vi "Periodic Tasks.vi"(8 "error in":errorcluster) -> ()   [LabVIEW 2015]
doc: "This VI runs in parallel to other tasks. It can contain as many user-defined periodic loops as you need. These can carry out PID or other sorts of timed response."
uses:
  <vilib>/Rock Robotics/Network Tables/NT Write Boolean.vi
  Robot Global Data.vi
  <vilib>/Rock Robotics/Network Tables/NT Write Numeric Array.vi
  <vilib>/Rock Robotics/Network Tables/NT Read Boolean.vi
  <vilib>/Rock Robotics/Network Tables/NT Write Number.vi
  <vilib>/Rock Robotics/SystemInterfaces/AI/FPGA_AIChannel.ctl
  Team900-VIs/navX Library v2/navX Library v2.lvlib
panel:
  out "Distance":bool
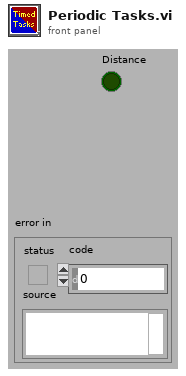
[diagram p1: front panel]
types:
  T1 = typedef "FPGA_AIChannel.ctl" = enum8{"AI 0", "AI 1", "AI 2", "AI 3", "AI MXP 0", "AI MXP 1", "AI MXP 2", "AI MXP 3", "Invalid"}
  T2 = typedef "WPI_AnalogChannelDevRef.ctl" = cluster{"DevStatus":errorcluster, "Analog Channel":T1}
  T3 = typedef "navX Library v2.lvlib/Z900_navX_DeviceTypeDef.ctl" = cluster{"Interface":cluster{"Protocol":T4, "Update Rate (4Hz-60Hz)":u8, "navX Open TypeDef":variant}, "Notify Packet":refnum<notifier>, "Loop VI Refnum":refnum<vi>, "Ready to Close Occurrence Refnum":refnum<k4>}
  T4 = typedef "navX Library v2.lvlib/Z900_navX_ProtocolTypeDef.ctl" = enum16{"SERIAL", "I2C", "SPI"}
  T5 = cluster{"Yaw":dbl, "Roll":dbl, "Pitch":dbl, "Heading":dbl, "Fused Heading":dbl}
  T6 = typedef "WPI_MotorControlDeviceRef.ctl" = cluster{"DeviceStatus":errorcluster, "Type":T7, "PWM":cluster{"PWM Channel":T8, "DeadBand":T9}, "CAN":cluster{"Device Number":u8, "Control Mode":T10, "Semaphore":T11, "Max Vout":dbl, "TalonSRX Control Mode":T12}, "Invert":bool}
  T7 = typedef "WPI_MotorControlType.ctl" = enum16{"PWM", "CAN", "CANTalonSRX"}
  T8 = typedef "FPGA_DIOPWMChannel.ctl" = enum8{"PWM 0", "PWM 1", "PWM 2", "PWM 3", "PWM 4", "PWM 5", "PWM 6", "PWM 7", "PWM 8", "PWM 9", "PWM MXP 0", "PWM MXP 1", "PWM MXP 2", "PWM MXP 3", "PWM MXP 4", "PWM MXP 5", "PWM MXP 6", "PWM MXP 7", "PWM MXP 8", "PWM MXP 9", "Invalid"}
  T9 = typedef "WPI_PWMDeadband.ctl" = cluster{"Name":string, "maxPositivePwm":i32, "minPositivePwm":i32, "centerPwm":i32, "maxNegativePwm":i32, "minNegativePwm":i32, "angularRange":u16}
  T10 = typedef "WPI_CANJaguar_ControlMode.ctl" = enum8{"Percent VBus", "Current", "Speed", "Position", "Voltage"}
  T11 = typedef "Semaphore RefNum" = refnum<k1>
  T12 = typedef "WPI_CANTalonSRX_APIControlMode.ctl" = enum8{"Percent VBus", "Speed", "Position", "Slave", "Unchanged / Invalid", "Voltage Compensation", "Current", "Motion Profile"}
  T13 = typedef "WPI_CANTalonSRX_GlobalStatus.ctl" = cluster{"Applied Throttle":dbl, "Module Enabled":bool, "CAN Error":errorcluster, "Closed Loop Error":dbl, "Forward Limit Switch Closed":bool, "Reverse Limit Switch Closed":bool, "Sensor Position":dbl, "Sensor Velocity":dbl, "Current":dbl, "Sticky Fault - Over Temp":bool, "Sticky Fault - Under Voltage":bool, "Sticky Fault - Forward Limit":bool, "Sticky Fault - Reverse Limit":bool, "Sticky Fault - Forward Soft Limit":bool, "Sticky Fault - Reverse Soft Limit":bool, "Brake is Enabled":bool, "Encoder Position":dbl, "Encoder Velocity":dbl, "Encoder Index Count":dbl, "Encoder A Pin State":bool, "Encoder B Pin State":bool, "Encoder Index Pin State":bool, "Analog In":dbl, "Analog In Velocity":dbl, "Temperature (C)":dbl, "Battery Voltage":dbl, "Control 5 Is Supported":bool, "Current Profile Slot Select":dbl, "Pos Div 8":bool, "Vel Div 4":bool, "Pulse Width Position":i32, "Pulse Width Velocity":i32, "Pulse Width Rise To Rise (us)":i32, "Pulse Width Rise To Fall (us)":i32, "Mot Prof Active Is Under Run":bool, "Mot Prof Active Has Under Run":bool, "Mot Prof Active Is Last":bool, "Mot Prof Active Velocity Only":bool, "Mot Prof Active Is Valid":bool, "Mot Prof Buffer Is Full":bool, "Mot Prof Active Profile Slot Select":i32, "Mot Prof NextID":i32, "Mot Prof Count":i32, "Mot Prof Active Velocity":dbl, "Mot Prof Active Position":dbl, "Mot Prof Output Enable":i32}
  T14 = typedef "WPI_DigitalInputDevRef.ctl" = cluster{"DevStatus":errorcluster, "DIO Channel":T15}
  T15 = typedef "FPGA_DIOChannel.ctl" = enum8{"DIO 0", "DIO 1", "DIO 2", "DIO 3", "DIO 4", "DIO 5", "DIO 6", "DIO 7", "DIO 8", "DIO 9", "DIO MXP 0", "DIO MXP 1", "DIO MXP 2", "DIO MXP 3", "DIO MXP 4", "DIO MXP 5", "DIO MXP 6", "DIO MXP 7", "DIO MXP 8", "DIO MXP 9", "DIO MXP 10", "DIO MXP 11", "DIO MXP 12", "DIO MXP 13", "DIO MXP 14", "DIO MXP 15", "Invalid"}
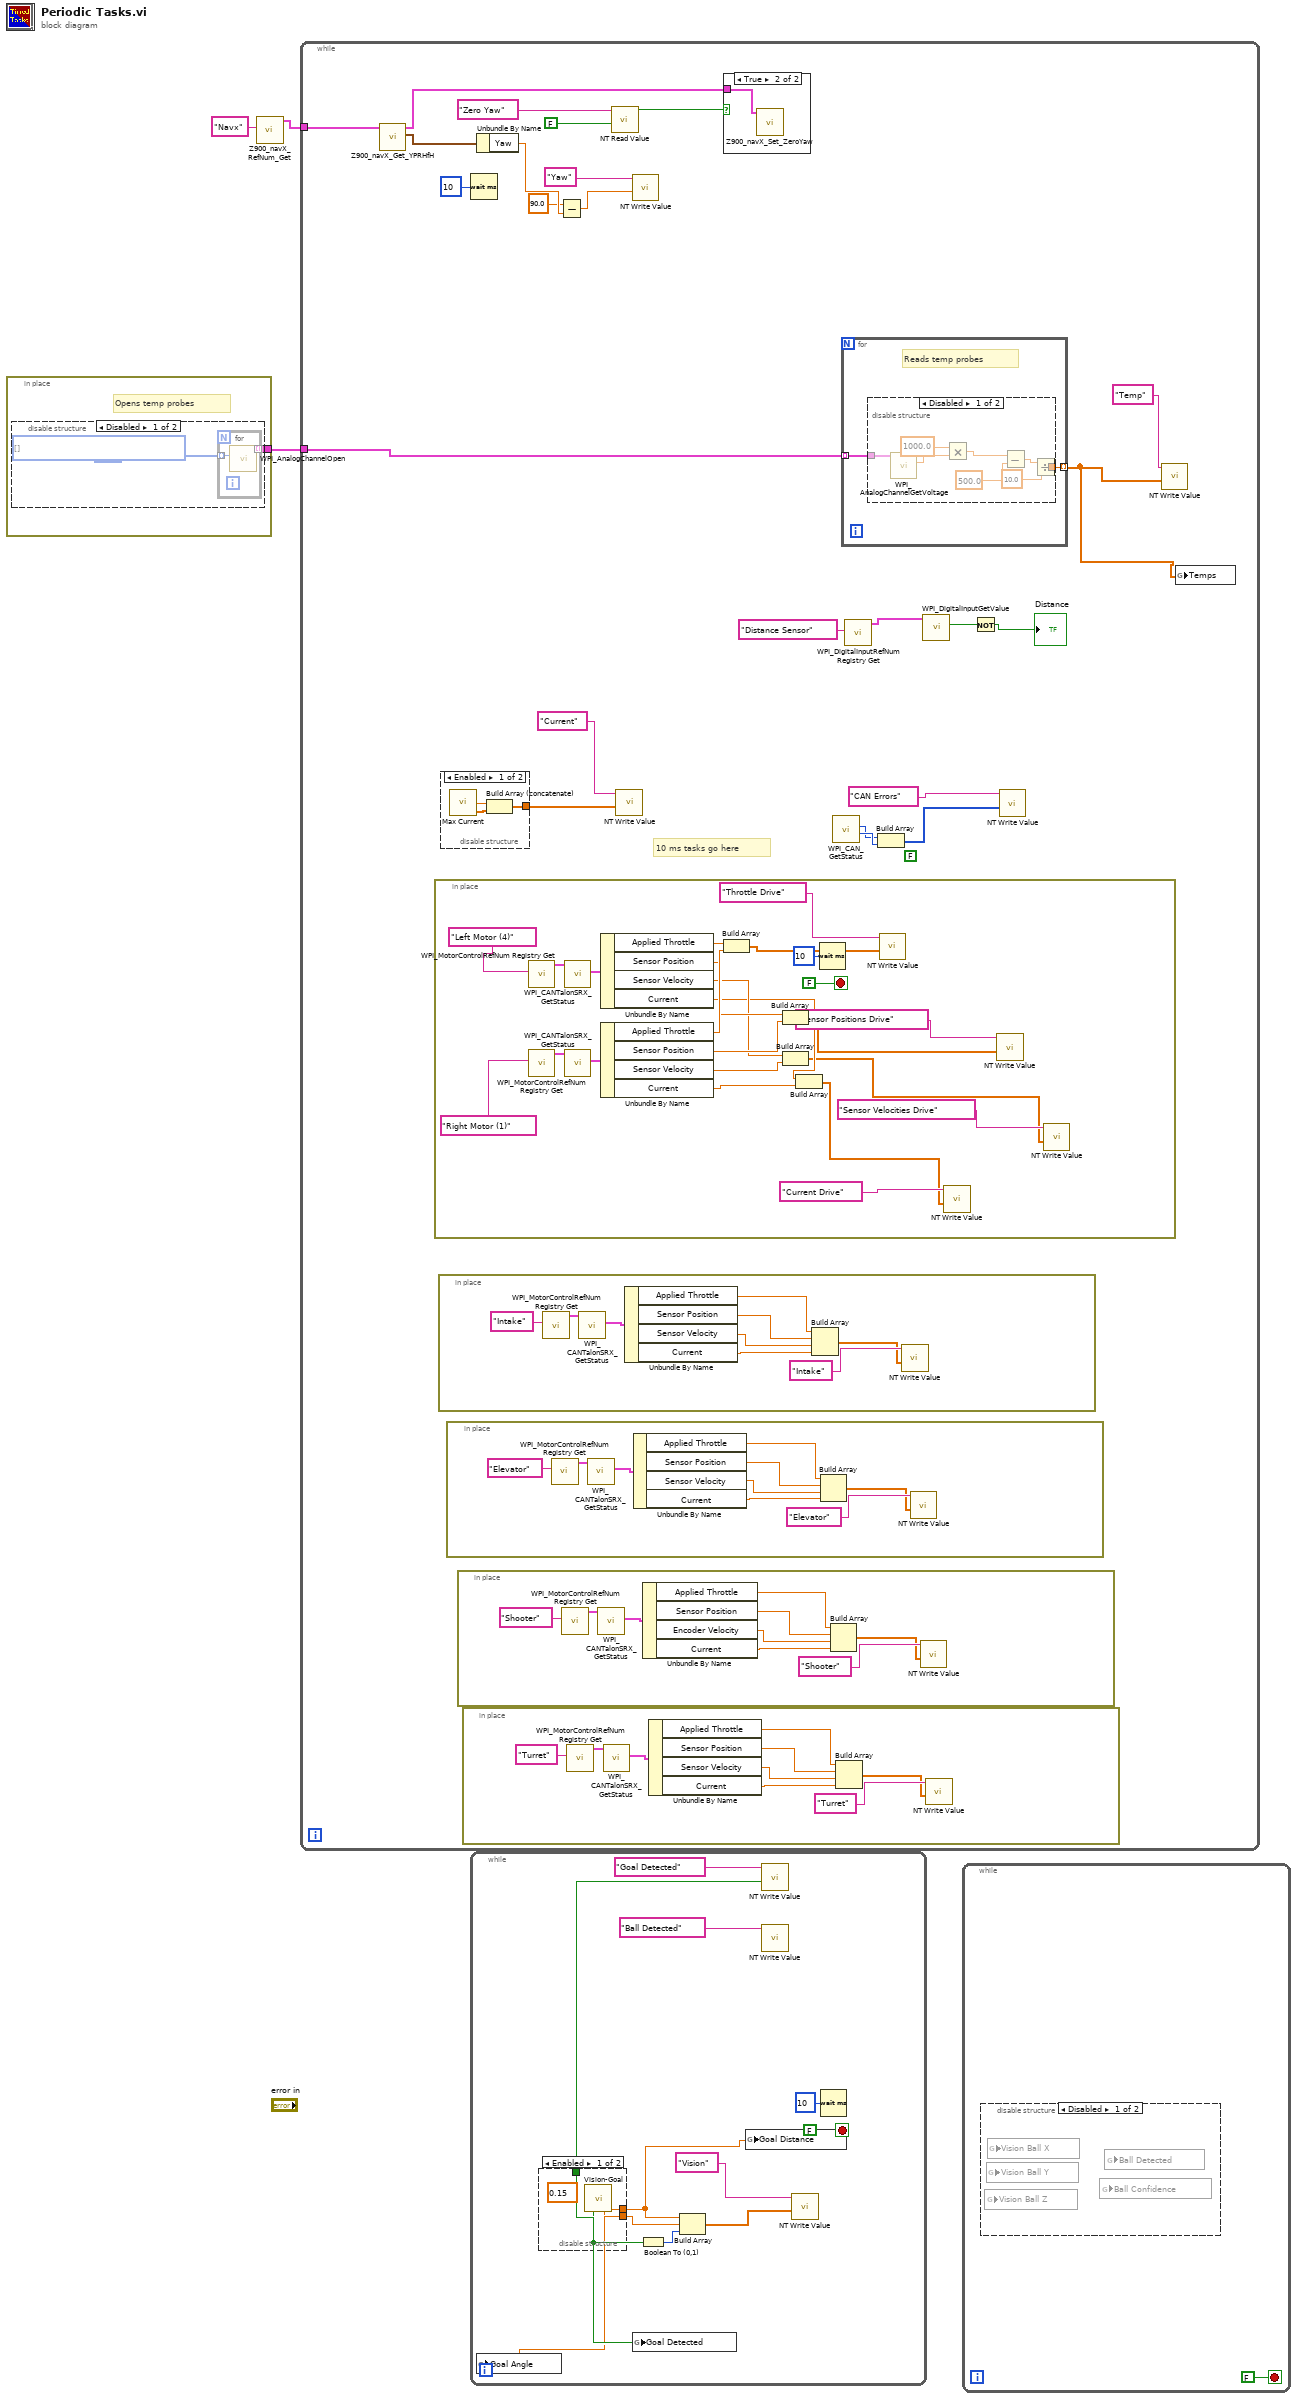
[diagram p0: block diagram]
diagram:
  n1 = in-place {
    in-place-border: [w4] -> w3
    # "Opens temp probes"
    n2 = disable-structure shown="Disabled" {
      disable-tunnel: [w5 _] -> w4
      frame Disabled {
        w6 = T1[] [] items=["AI 0", "AI 1", "AI 2", "AI 3", "AI MXP 0", "AI MXP 1", "AI MXP 2", "AI MXP 3", "Invalid"] ("Analog Channel")
        n3 = for {
          tunnel: w6 -> [w8] mode=indexing
          tunnel: [w7] -> w5 mode=indexing
          n4 = call <vilib>:"WPI_AnalogChannelOpen.vi"("Analog Channel"=w8) -> ("AIDeviceRef"=w7:T2)  [unwired: 9 in, 1 out]
        }
      }
      frame Enabled {
      }
    }
  }
  n5 = call "Z900_navX_RefNum_Get.vi"("refnum name"="Navx") -> ("navX Device"=w1:T3)  [unwired: 9 in, 1 out]
  n6 = while {
    tunnel: w3 -> [w14]
    tunnel: w1 -> [w20]
    stop <- FALSE stop-if-true
    (unwired) FALSE
    # "10 ms tasks go here"
    n7 = call "Z900_navX_Get_YPRHfH.vi"("navX Device"=w20) -> ("YRPHfH"=w19:T5, "navX Device"=w18:T3)  [unwired: 7 in, 2 out]
    n8 = in-place {
      n9 = call <vilib>:"WPI_MotorControlRefNum Registry Get.vi"("refnum name"="Left Motor (4)") -> ("MotorControlDevRef"=w101:T6)  [unwired: 9 in, 1 out]
      n10 = call <vilib>:"WPI_MotorControlRefNum Registry Get.vi"("refnum name"="Right Motor (1)") -> ("MotorControlDevRef"=w102:T6)  [unwired: 9 in, 1 out]
      n11 = call <vilib>:"WPI_CANTalonSRX_GetStatus.vi"("CAN Talon SRX Ref"=w101) -> ("Talon SRX Status"=w99:T13)  [unwired: 8 in, 2 out]
      n12 = call <vilib>:"WPI_CANTalonSRX_GetStatus.vi"("CAN Talon SRX Ref"=w102) -> ("Talon SRX Status"=w100:T13)  [unwired: 8 in, 2 out]
      n13 = Unbundle By Name(w99) -> ("Applied Throttle"=w98:dbl, "Sensor Position"=w96:dbl, "Sensor Velocity"=w94:dbl, "Current"=w91:dbl)
      n14 = Unbundle By Name(w100) -> ("Applied Throttle"=w97:dbl, "Sensor Position"=w95:dbl, "Sensor Velocity"=w93:dbl, "Current"=w92:dbl)
      n15 = Build Array(w98, w97) -> (w89:dbl[])
      n16 = Build Array(w96, w95) -> (w87:dbl[])
      n17 = Build Array(w94, w93) -> (w85:dbl[])
      n18 = Build Array(w91, w92) -> (w83:dbl[])
      n19 = call-poly <vilib>:"NT Write Value.vi"("Numeric Array"=w89, "Name"="Throttle Drive") -> ()  [unwired: 9 in, 1 out]
      n20 = call-poly <vilib>:"NT Write Value.vi"("Numeric Array"=w83, "Name"="Current Drive") -> ()  [unwired: 9 in, 1 out]
      n21 = call-poly <vilib>:"NT Write Value.vi"("Numeric Array"=w87, "Name"="Sensor Positions Drive") -> ()  [unwired: 9 in, 1 out]
      n22 = call-poly <vilib>:"NT Write Value.vi"("Numeric Array"=w85, "Name"="Sensor Velocities Drive") -> ()  [unwired: 9 in, 1 out]
    }
    n23 = in-place {
      n24 = call <vilib>:"WPI_MotorControlRefNum Registry Get.vi"("refnum name"="Intake") -> ("MotorControlDevRef"=w79:T6)  [unwired: 9 in, 1 out]
      n25 = call <vilib>:"WPI_CANTalonSRX_GetStatus.vi"("CAN Talon SRX Ref"=w79) -> ("Talon SRX Status"=w78:T13)  [unwired: 8 in, 2 out]
      n26 = Unbundle By Name(w78) -> ("Applied Throttle"=w77:dbl, "Sensor Position"=w76:dbl, "Sensor Velocity"=w75:dbl, "Current"=w74:dbl)
      n27 = Build Array(w77, w76, w75, w74) -> (w72:dbl[])
      n28 = call-poly <vilib>:"NT Write Value.vi"("Numeric Array"=w72, "Name"="Intake") -> ()  [unwired: 9 in, 1 out]
    }
    n29 = disable-structure shown="Enabled" {
      disable-tunnel: [w103 _] -> w27
      frame Enabled {
        n30 = call "Max Current.vi"() -> ("Currents By Channel"=w104:dbl[], "Current"=w105:dbl)  [unwired: 1 out]
        n31 = Build Array (concatenate)(w105, w104) -> (w103:dbl[])
      }
      frame Disabled {
      }
    }
    n32 = in-place {
      n33 = call <vilib>:"WPI_MotorControlRefNum Registry Get.vi"("refnum name"="Elevator") -> ("MotorControlDevRef"=w70:T6)  [unwired: 9 in, 1 out]
      n34 = call <vilib>:"WPI_CANTalonSRX_GetStatus.vi"("CAN Talon SRX Ref"=w70) -> ("Talon SRX Status"=w69:T13)  [unwired: 8 in, 2 out]
      n35 = Unbundle By Name(w69) -> ("Applied Throttle"=w68:dbl, "Sensor Position"=w67:dbl, "Sensor Velocity"=w66:dbl, "Current"=w65:dbl)
      n36 = Build Array(w68, w67, w66, w65) -> (w63:dbl[])
      n37 = call-poly <vilib>:"NT Write Value.vi"("Numeric Array"=w63, "Name"="Elevator") -> ()  [unwired: 9 in, 1 out]
    }
    n38 = in-place {
      n39 = call <vilib>:"WPI_MotorControlRefNum Registry Get.vi"("refnum name"="Shooter") -> ("MotorControlDevRef"=w61:T6)  [unwired: 9 in, 1 out]
      n40 = call <vilib>:"WPI_CANTalonSRX_GetStatus.vi"("CAN Talon SRX Ref"=w61) -> ("Talon SRX Status"=w60:T13)  [unwired: 8 in, 2 out]
      n41 = Unbundle By Name(w60) -> ("Applied Throttle"=w59:dbl, "Sensor Position"=w58:dbl, "Encoder Velocity"=w57:dbl, "Current"=w56:dbl)
      n42 = Build Array(w59, w58, w57, w56) -> (w54:dbl[])
      n43 = call-poly <vilib>:"NT Write Value.vi"("Numeric Array"=w54, "Name"="Shooter") -> ()  [unwired: 9 in, 1 out]
    }
    n44 = in-place {
      n45 = call <vilib>:"WPI_MotorControlRefNum Registry Get.vi"("refnum name"="Turret") -> ("MotorControlDevRef"=w52:T6)  [unwired: 9 in, 1 out]
      n46 = call <vilib>:"WPI_CANTalonSRX_GetStatus.vi"("CAN Talon SRX Ref"=w52) -> ("Talon SRX Status"=w51:T13)  [unwired: 8 in, 2 out]
      n47 = Unbundle By Name(w51) -> ("Applied Throttle"=w50:dbl, "Sensor Position"=w49:dbl, "Sensor Velocity"=w48:dbl, "Current"=w47:dbl)
      n48 = Build Array(w50, w49, w48, w47) -> (w45:dbl[])
      n49 = call-poly <vilib>:"NT Write Value.vi"("Numeric Array"=w45, "Name"="Turret") -> ()  [unwired: 9 in, 1 out]
    }
    n50 = Wait (ms)(milliseconds to wait=u32 10) -> ()  [unwired: 1 out]
    n51 = Unbundle By Name(w19) -> ("Yaw"=w17:dbl)
    n52 = Subtract(x=90.0, y=w17) -> (x-y=w16:dbl)
    n53 = call-poly <vilib>:"NT Read Value.vi"("Default Value"=FALSE, "Name"="Zero Yaw") -> ("Boolean"=w31:bool)  [unwired: 8 in, 1 out]
    n54 = call-poly <vilib>:"NT Write Value.vi"("Numeric Array"=w27, "Name"="Current") -> ()  [unwired: 9 in, 1 out]
    n55 = call-poly <vilib>:"NT Write Value.vi"("Numeric"=w16, "Name"="Yaw") -> ()  [unwired: 9 in, 1 out]
    n56 = case shown="True" w31 {
      tunnel: w18 -> [_ w106]
      frame False {
      }
      frame True {
        n57 = call "Z900_navX_Set_ZeroYaw.vi"("navX Device"=w106) -> ()  [unwired: 9 in, 2 out]
      }
    }
    n58 = Wait (ms)(milliseconds to wait=u32 10) -> ()  [unwired: 1 out]
    n59 = call <vilib>:"WPI_CAN_GetStatus.vi"() -> ("Transmit Error Count"=w24:u32, "Receive Error Count"=w23:u32)  [unwired: 6 in, 4 out]
    n60 = for {
      tunnel: w14 -> [w36] mode=indexing
      tunnel: [w35] -> w21 mode=indexing
      # "Reads temp probes"
      n61 = disable-structure shown="Disabled" {
        disable-tunnel: w36 -> [w44 _]
        disable-tunnel: [w37 _] -> w35
        frame Disabled {
          n62 = call <vilib>:"WPI_AnalogChannelGetVoltage.vi"("AIDeviceRef"=w44) -> ("Voltage"=w40:dbl)  [unwired: 8 in, 2 out]
          n63 = Multiply(x=1000.0, y=w40) -> (x*y=w38:dbl)
          n64 = Subtract(x=w38, y=500.0) -> (x-y=w42:dbl)
          n65 = Divide(x=w42, y=10.0) -> (x/y=w37:dbl)
        }
        frame Enabled {
        }
      }
    }
    n66 = call <vilib>:"WPI_DigitalInputRefNum Registry Get.vi"("refnum name"="Distance Sensor") -> ("DigitalInputDevRef"=w12:T14)  [unwired: 9 in, 1 out]
    n67 = Build Array(w23, w24) -> (w25:u32[])
    n68 = call <vilib>:"WPI_DigitalInputGetValue.vi"("DigitalInputDevRef"=w12) -> ("Value"=w10:bool)  [unwired: 8 in, 2 out]
    n69 = Not(x=w10) -> (.not. x?=→"Distance":bool)
    n70 = call-poly <vilib>:"NT Write Value.vi"("Numeric Array"=w25, "Name"="CAN Errors") -> ()  [unwired: 9 in, 1 out]
    n71 = call-poly <vilib>:"NT Write Value.vi"("Numeric Array"=w21, "Name"="Temp") -> ()  [unwired: 9 in, 1 out]
    n72 = global write "Robot Global Data.vi" "Temps"(w21) -> ()
  }
  n73 = while {
    stop <- FALSE stop-if-true
    n74 = disable-structure shown="Enabled" {
      disable-tunnel: [w119 _] -> w109
      disable-tunnel: [w118 _] -> w108
      disable-tunnel: [w117 _] -> w107
      frame Enabled {
        (unwired) 0.15 ("Minimum Confidence")
        n75 = call "Vision-Goal.vi"() -> ("Goal Detected"=w119:bool, "Goal Angle (radians 0=right)"=w117:dbl, "Goal Distance (from front of shooter)"=w118:dbl)  [unwired: 13 in]
      }
      frame Disabled {
      }
    }
    n76 = global write "Robot Global Data.vi" "Goal Angle"(w107) -> ()
    n77 = global write "Robot Global Data.vi" "Goal Detected"(w109) -> ()
    n78 = Boolean To (0,1)(Boolean=w109) -> (0, 1=w110:i16)
    n79 = Build Array(w108, w107, w110) -> (w111:dbl[])
    n80 = global write "Robot Global Data.vi" "Goal Distance"(w108) -> ()
    n81 = call-poly <vilib>:"NT Write Value.vi"("Boolean"=w109, "Name"="Goal Detected") -> ()  [unwired: 9 in, 1 out]
    n82 = call-poly <vilib>:"NT Write Value.vi"("Name"="Ball Detected") -> ()  [unwired: 10 in, 1 out]
    n83 = call-poly <vilib>:"NT Write Value.vi"("Numeric Array"=w111, "Name"="Vision") -> ()  [unwired: 9 in, 1 out]
    n84 = Wait (ms)(milliseconds to wait=u32 10) -> ()  [unwired: 1 out]
  }
  n85 = while {
    stop <- FALSE stop-if-true
    n86 = disable-structure shown="Disabled" {
      frame Disabled {
        n87 = global read "Robot Global Data.vi" "Vision Ball Z"() -> ()  [unwired: 1 in]
        n88 = global read "Robot Global Data.vi" "Vision Ball Y"() -> ()  [unwired: 1 in]
        n89 = global read "Robot Global Data.vi" "Vision Ball X"() -> ()  [unwired: 1 in]
        n90 = global read "Robot Global Data.vi" "Ball Confidence"() -> ()  [unwired: 1 in]
        n91 = global read "Robot Global Data.vi" "Ball Detected"() -> ()  [unwired: 1 in]
      }
      frame Enabled {
      }
    }
  }
